vi "Auto Index_winding.vi"(10 "Recipes.Winding":T2(array[cluster])) -> (2 "Array":T1(array[cluster]))   [LabVIEW 2014]
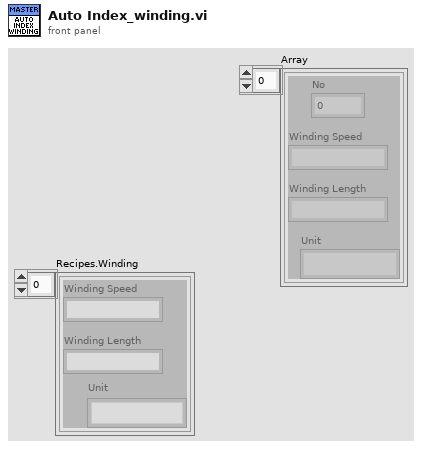
[diagram p1: front panel]
types:
  T1 = cluster{"No":dbl, "Winding Speed":string, "Winding Length":string, "Unit":string}[]
  T2 = cluster{"Winding Speed":string, "Winding Length":string, "Unit":string}[]
  T3 = cluster{"No":dbl, "Winding Speed":string, "Winding Length":string, "Unit":string}
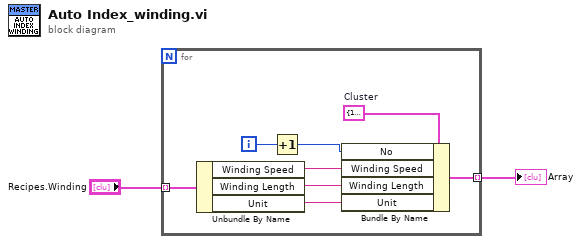
[diagram p0: block diagram]
diagram:
  n1 = for {
    tunnel: "Recipes.Winding" -> [w10] mode=indexing
    tunnel: [w5] -> w1 mode=indexing
    i -> [w3]
    w9 = T3 {"No"=1.0, "Winding Speed"="", "Winding Length"="", "Unit"="mm"}  # Cluster
    n2 = Unbundle By Name(w10) -> ("Winding Speed"=w8:string, "Winding Length"=w7:string, "Unit"=w6:string)
    n3 = Increment(x=w3) -> (x+1=w4:i32)
    n4 = Bundle By Name(cluster=w9, "No"=w4, "Winding Speed"=w8, "Winding Length"=w7, "Unit"=w6) -> (w5:T3)
  }
  "Array" <- w1
